vi "9239_2.vi"() -> ()   [LabVIEW 2014]
uses:
  <vilib>/Platform/TimedLoop/XDataNode/timing_clust.ctl
  <vilib>/Platform/TimedLoop/XDataNode/nitl_modes.ctl
  <vilib>/Platform/TimedLoop/XDataNode/wakeup.ctl
  <vilib>/Platform/TimedLoop/XDataNode/XDataNode.xnode
  <vilib>/Platform/TimedLoop/XDataNode/XDNodeRunTimeDep.lvlib
  <vilib>/Analysis/NI_AALBase.lvlib
panel:
  out "ai1标准差":dbl
  out "ai2标准差":dbl
  out "ai2通道零漂采集 2":dynamicdata(graph)
  out "已采样数量":dbl
  out "ai1通道零漂采集":dynamicdata(graph)
  out "数据记录频率":dbl
  in  "路径":path
  in  "采样数":dbl=2000.0
  in  "采样率":dbl=2000.0
  out "时间":string
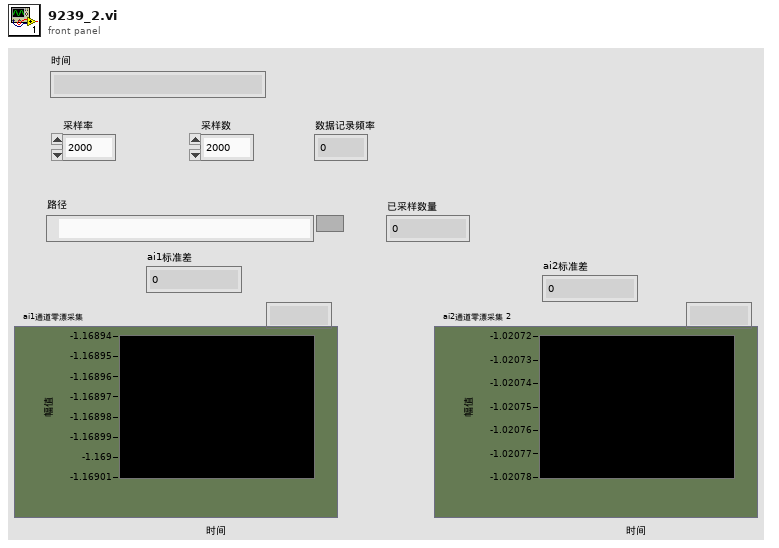
[diagram p1: front panel]
types:
  T1 = enum16{"open", "open or create", "create or replace", "create", "open (read-only)"}
  T2 = typedef "XDNodeRunTimeDep.lvlib/timing_clust.ctl" = cluster{"Expected End [f-1]":u64, "Actual End [f-1]":u64, "Finished Late? [f-1]":bool, "Expected End [i-1]":u64, "Actual End [i-1]":u64, "Finished Late? [i-1]":bool, "Expected Start [i]":u64, "Actual Start [i]":u64, "Expected Start [f]":u64, "Actual Start [f]":u64, "Source Name":string, "Structure Name":string, "Period":i64, "Deadline":i64, "Offset":i64, "Start":i64, "Priority":i32, "Timeout":i32, "Mode":T3, "Wakeup Reason":T4, "Error":errorcluster, "Source Type":string, "Secondary Source Type":string, "Global End Time":u64, "Global Start Time":u64, "Frame Duration":u64, "Iteration Duration":u64, "Assigned CPU":i32, "I/O Scan Engine Mode":u32}
  T3 = typedef "XDNodeRunTimeDep.lvlib/nitl_modes.ctl" = enum32{"No Change", "Process missed periods, maintain original phase", "Discard missed periods, maintain original phase", "Process missed periods, ignore original phase", "Discard missed periods, ignore original phase"}
  T4 = typedef "XDNodeRunTimeDep.lvlib/wakeup.ctl" = enum32{"Normal", "Aborted", "Asynchronous wakeup", "Timing source error", "Timed loop error", "Timeout"}
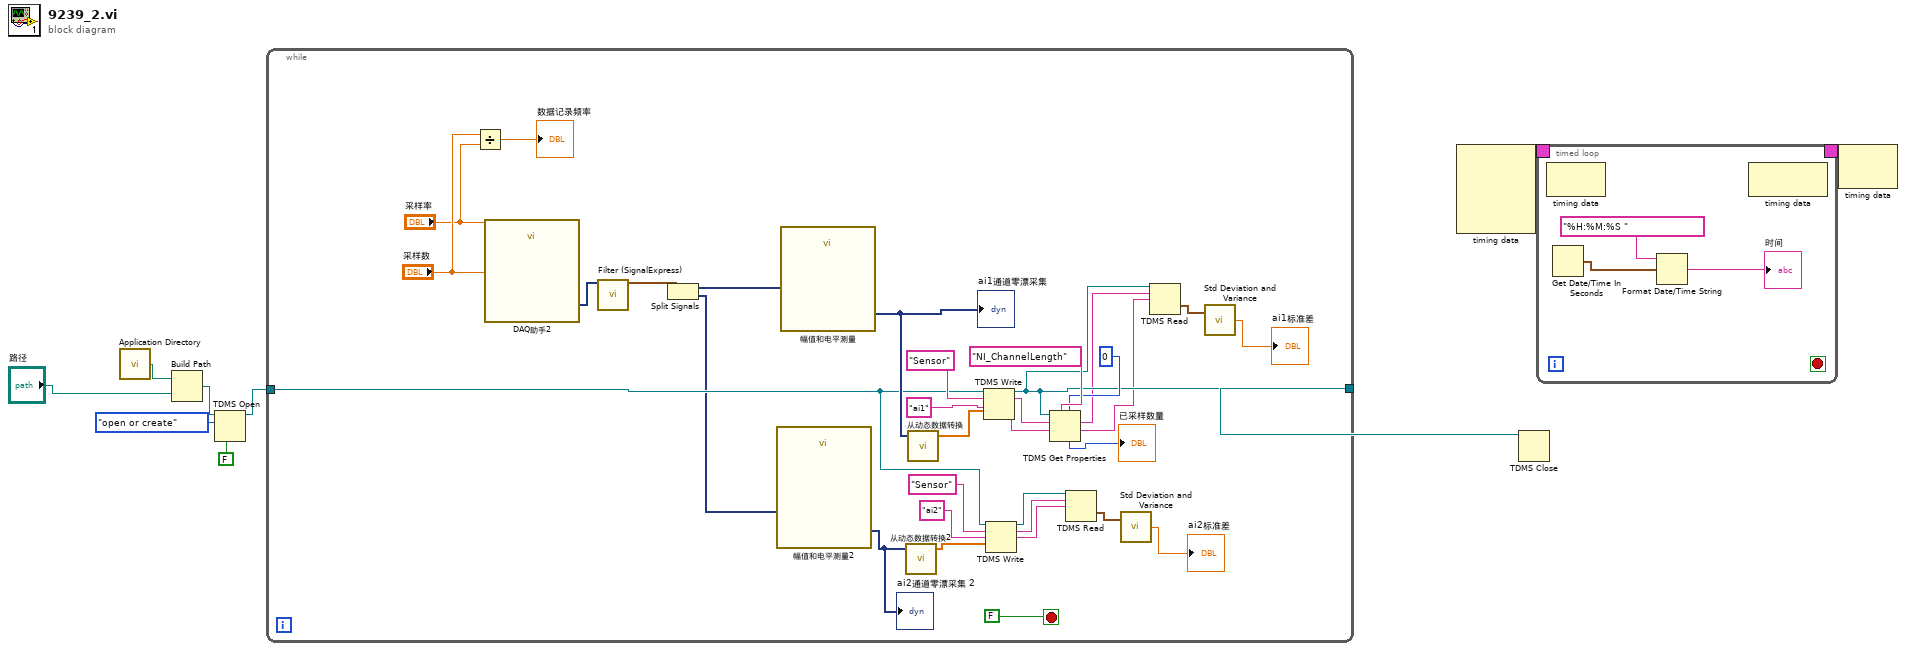
[diagram p0: block diagram]
diagram:
  n1 = call <vilib>:"Application Directory.vi"() -> ("Application Directory"=w2:path)
  n2 = Build Path(base path=w2, name or relative path="路径") -> (appended path=w6:path)
  n3 = TDMS Open(6:FALSE ("disable buffering (T)"), 10:T1."open or create" ("operation"), 11:w6) -> (3:w4:refnum<k34>)  [unwired: 4 in, 1 out]
  n4 = while {
    tunnel: w4 -> [w25]
    tunnel: [w13] -> w1
    stop <- FALSE stop-if-true
    n5 = Divide(x="采样数", y="采样率") -> (x/y=→"数据记录频率":dbl)
    n6 = call "DAQ助手2"("速率"="采样率", "采样数"="采样数") -> ("data"=w37:dynamicdata)  [unwired: 14 in, 3 out]
    n7 = call "Filter (SignalExpress)"("input signals"=w37) -> ("filtered data"=w36:waveform(dbl)[])  [unwired: 17 in, 1 out]
    n8 = Split Signals(w36) -> (w21:dynamicdata, w16:dynamicdata)  [unwired: 2 in]
    n9 = call "幅值和电平测量2"("Signals"=w16) -> ("Mean (DC)"=w24:dynamicdata)  [unwired: 13 in, 1 out]
    "ai2通道零漂采集 2" <- w24
    n10 = call "幅值和电平测量"("Signals"=w21) -> ("Mean (DC)"=w33:dynamicdata)  [unwired: 13 in, 1 out]
    "ai1通道零漂采集" <- w33
    n11 = call "从动态数据转换2"("Dynamic Data Type"=w24) -> ("Array"=w22:dbl[])  [unwired: 3 in]
    n12 = call "从动态数据转换"("Dynamic Data Type"=w33) -> ("Array"=w23:dbl[])  [unwired: 3 in]
    n13 = TDMS Write(0:w25, 5:"Sensor", 7:"ai1", 9:w23) -> (4:w13:refnum<k34>, 6:w32:string, 8:w31:string)  [unwired: 2 in, 1 out]
    n14 = TDMS Write(0:w25, 5:"Sensor", 7:"ai2", 9:w22) -> (4:w20:refnum<k34>, 6:w19:string, 8:w18:string)  [unwired: 2 in, 1 out]
    n15 = TDMS Get Properties(5:0, 7:"NI_ChannelLength", 9:w31, 10:w32, 11:w13) -> (1:w11:string, 2:w12:string, 4:→"已采样数量":i32)  [unwired: 1 in, 3 out]
    n16 = TDMS Read(0:w20, 5:w19, 7:w18) -> (10:w17:waveform(dbl))  [unwired: 5 in, 5 out]
    n17 = call <vilib>:"Std Deviation and Variance.vi"("X"=w17) -> ("standard deviation"=→"ai2标准差":dbl)  [unwired: 1 in, 2 out]
    n18 = TDMS Read(0:w13, 5:w12, 7:w11) -> (10:w15:waveform(dbl))  [unwired: 5 in, 5 out]
    n19 = call <vilib>:"Std Deviation and Variance.vi"("X"=w15) -> ("standard deviation"=→"ai1标准差":dbl)  [unwired: 1 in, 2 out]
  }
  n20 = node-c288() -> (w9:T2)  [unwired: 4 in]
  n21 = TDMS Close(11:w1) -> ()  [unwired: 1 in, 2 out]
  n22 = timed-loop {
    timing: w9 -> [_]
    timing-out: [_] -> w8
    stop <- _ stop-if-true
    n23 = node-c288() -> ()  [unwired: 1 in, 1 out]
    n24 = Get Date/Time In Seconds() -> (seconds since 1Jan1904=w44:timestamp)
    n25 = Format Date/Time String(time format string (%c)="%H:%M:%S ", seconds (now)=w44) -> (date/time string=→"时间":string)  [unwired: 1 in]
    n26 = node-c288() -> ()  [unwired: 1 in, 1 out]
  }
  n27 = node-c288(w8) -> ()  [unwired: 1 out]
